vi "DefBallEnemySkill.vi"(8 "error in (no error)":errorcluster, 9 "Robot":refnum<class "Robot.lvclass">, 10 "Game":refnum<class "Game.lvclass">, 11 "DefBallEnemySkill in":refnum<class "DefBallEnemySkill.lvclass">) -> (0 "error out":errorcluster, 2 "robot out":refnum<class "Robot.lvclass">, 3 "DefBallEnemySkill out":refnum<class "DefBallEnemySkill.lvclass">)   [LabVIEW 2018, in "DefBallEnemySkill.lvclass"]
uses:
  DefBallEnemySkill.lvclass
  Robot_class/Robot.lvclass
  C:/Users/Ronaldo/Desktop/Phoenix/SSL_AI/Object_class/Object.lvclass
  Game_class/Game.lvclass
  Utilities_class/Utilities.lvclass
  Game_class/Game.lvclass/Game.ctl
  Object_class/Object.lvclass/Object.ctl
  Robot_class/Robot.lvclass/Robot.ctl
  Game_class/Read BallRef.vi
  Object_class/Read x.vi
  Object_class/Read y.vi
  Game_class/Read FieldRef.vi
  Game_class/Read Utilities.lvclass.vi
  Robot_class/Write dest_x.vi
  Robot_class/Write dest_y.vi
  Robot_class/Write dest_orientation.vi
  Ball_class/Ball.lvclass
  Field_class/Field.lvclass
panel:
  in  "goalie distance from goal line":dbl=150.0
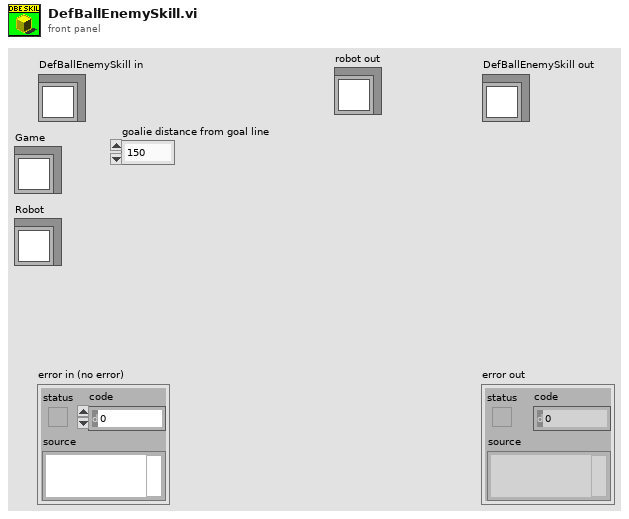
[diagram p1: front panel]
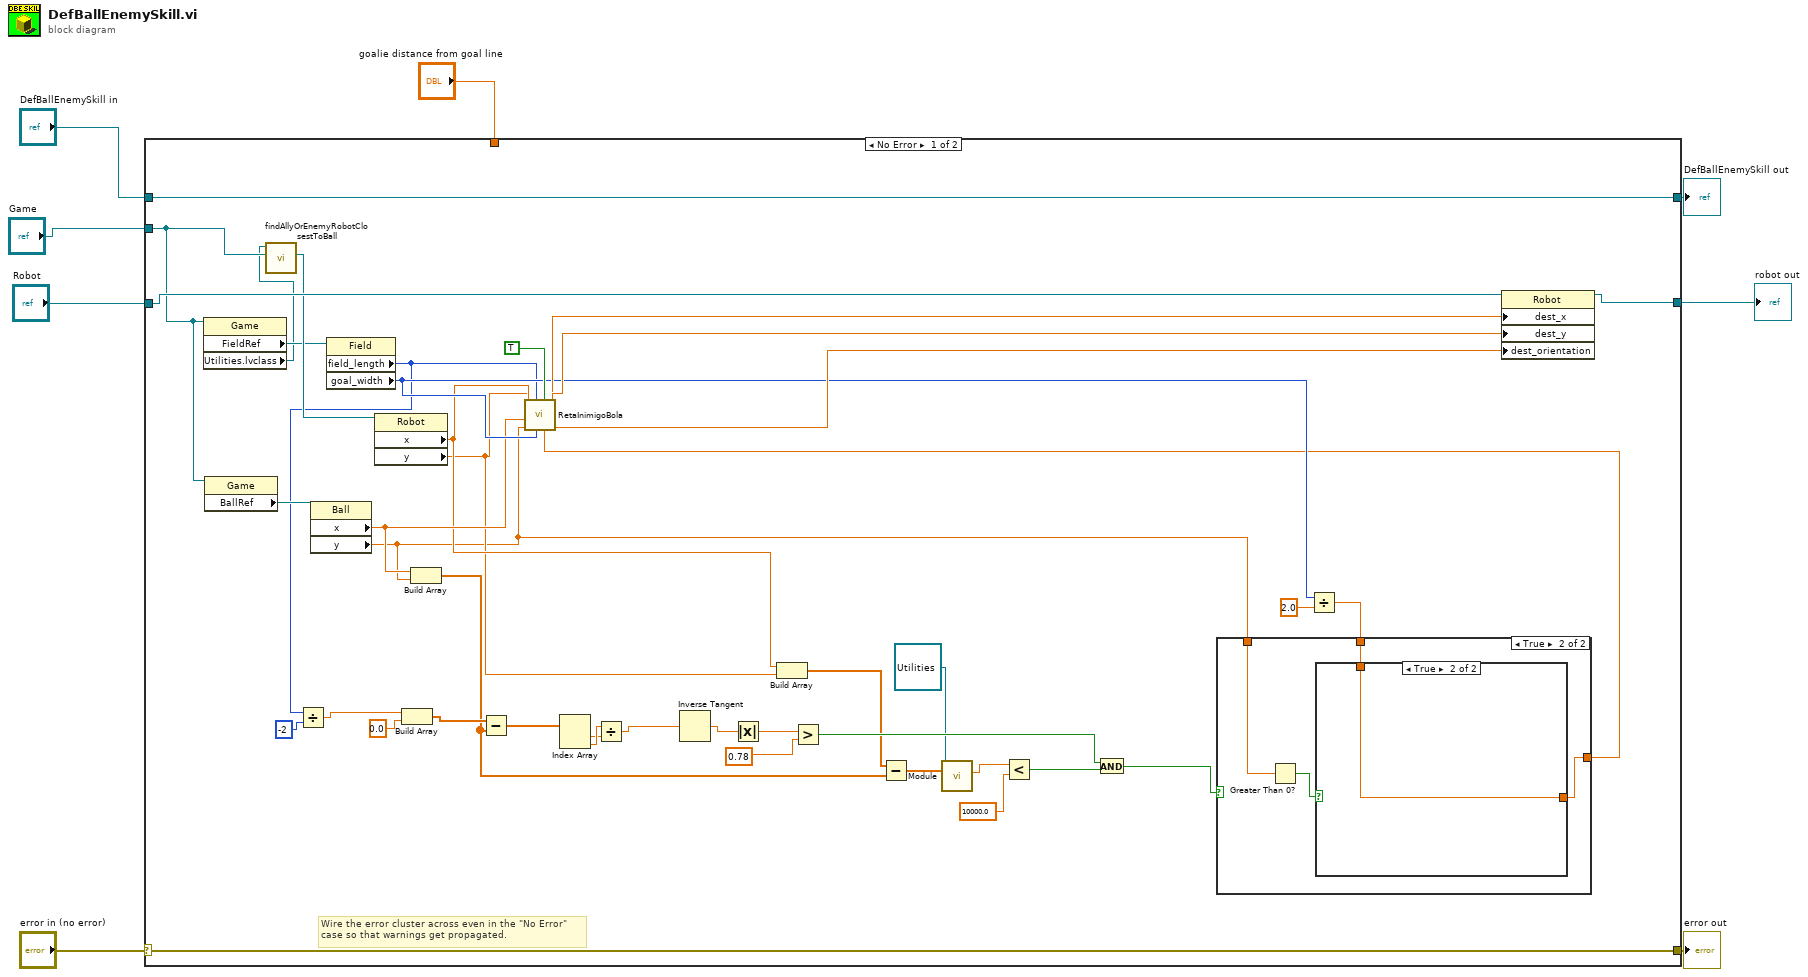
[diagram p0: block diagram]
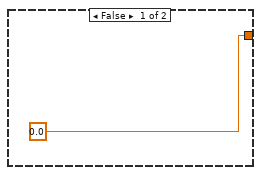
[diagram p2: hidden frame]
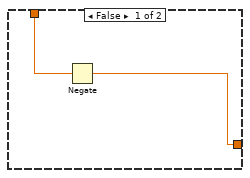
[diagram p3: hidden frame]
diagram:
  n1 = case shown="No Error" "error in (no error)" {
    selector: "error in (no error)" -> [w49 w60]
    tunnel: [w49 w60] -> w7
    tunnel: [w50 w59] -> w5
    tunnel: "DefBallEnemySkill in" -> [w50 w59]
    tunnel: "Robot" -> [w48 _]
    tunnel: "Game" -> [w46 _]
    tunnel: "goalie distance from goal line" -> [_ _]
    tunnel: [w10 _] -> w1
    frame No Error {
      # "Wire the error cluster across even in the \"No Error\"\ncase so that warnings get propagated."
      n2 = property class="Game"(reference=w46) -> ("FieldRef"=w44:refnum<class "Field.lvclass">, "Utilities.lvclass"=w12:refnum<class "Utilities.lvclass">)  [unwired: 1 in, 2 out]
      n3 = property class="Game"(reference=w46) -> ("BallRef"=w45:refnum<class "Ball.lvclass">)  [unwired: 1 in, 2 out]
      n4 = call "findAllyOrEnemyRobotClosestToBall.vi"("Game"=w46, "Utilities in"=w12) -> ("Robot"=w47:refnum<class "Robot.lvclass">)  [unwired: 6 in, 3 out]
      n5 = property class="Ball"(reference=w45) -> ("x"=w24:dbl, "y"=w11:dbl)  [unwired: 1 in, 2 out]
      n6 = property class="Field"(reference=w44) -> ("field_length"=w25:i32, "goal_width"=w37:i32)  [unwired: 1 in, 2 out]
      n7 = Divide(x=w25, y=-2) -> (x/y=w31:dbl)
      n8 = property class="Robot"(reference=w47) -> ("x"=w17:dbl, "y"=w16:dbl)  [unwired: 1 in, 2 out]
      n9 = Build Array(w31, 0.0 ("element")) -> (w34:dbl[])
      n10 = Build Array(w24, w11) -> (w14:dbl[])
      n11 = Subtract(x=w34, y=w14) -> (x-y=w33:dbl[])
      n12 = Index Array(array=w33) -> (element #1=w29:dbl, element #2=w30:dbl)  [unwired: 2 in]
      n13 = Divide(x=w30, y=w29) -> (x/y=w28:dbl)
      n14 = Inverse Tangent(1:w28) -> (0:w27:dbl)
      n15 = Absolute Value(x=w27) -> (abs(x)=w32:dbl)
      n16 = Build Array(w17, w16) -> (w15:dbl[])
      n17 = Greater?(x=w32, y=0.78) -> (0:w21:bool)
      n18 = Subtract(x=w15, y=w14) -> (x-y=w19:dbl[])
      n19 = call-dynamic "Module.vi"("2D vector"=w19, "Utilities in"=refnum<class "Utilities.lvclass"> refnum) -> ("Modulo"=w18:dbl)  [unwired: 7 in, 2 out]
      n20 = Less?(x=w18, y=10000.0) -> (x < y?=w22:bool)
      n21 = And(x=w21, y=w22) -> (x .and. y?=w20:bool)
      n22 = Divide(x=w37, y=2.0) -> (x/y=w39:dbl)
      n23 = case shown="True" w20 {
        tunnel: w39 -> [_ w54]
        tunnel: [0.0 w53] -> w13
        tunnel: w11 -> [_ w52]
        frame False {
        }
        frame True {
          n24 = Greater Than 0?(x=w52) -> (x > 0?=w55:bool)
          n25 = case shown="True" w55 {
            tunnel: w54 -> [w57 w58]
            tunnel: [w56 w58] -> w53
            frame False {
              n26 = Negate(x=w57) -> (-x=w56:dbl)
            }
            frame True {
            }
          }
        }
      }
      n27 = call "RetaInimigoBola.vi"("Y quina"=w13, "Meio?"=TRUE, "Goal width"=w37, "Field lenght"=w25, "Y bola"=w11, "X bola"=w24, "Y inimigo"=w16, "X inimigo"=w17) -> ("Orientação"=w41:dbl, "Y goleiro"=w43:dbl, "X goleiro"=w42:dbl)  [unwired: 1 in]
      n28 = property class="Robot"(reference=w48, "dest_x"=w42, "dest_y"=w43, "dest_orientation"=w41) -> (reference out=w10:refnum<class "Robot.lvclass">)  [unwired: 1 in, 1 out]
    }
    frame Error {
    }
  }
  "error out" <- w7
  "DefBallEnemySkill out" <- w5
  "robot out" <- w1
